vi "New One-Shot Subscription.vi"(10 "Ignore Past Updates? (F)":bool, 11 "OneShotSubscription In":refnum<class "OneShotSubscription.lvclass">) -> (3 "OneShotSubscription Out":refnum<class "OneShotSubscription.lvclass">)   [LabVIEW 2015, in "Mediator.lvlib" / "OneShotSubscription.lvclass"]
uses:
  OneShotSubscription.lvclass
  OneShotSubscription.lvclass/OneShotSubscription.ctl
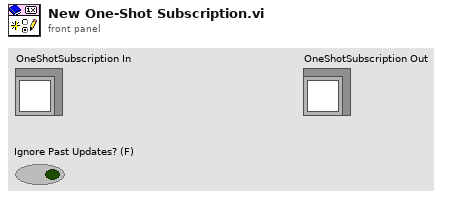
[diagram p1: front panel]
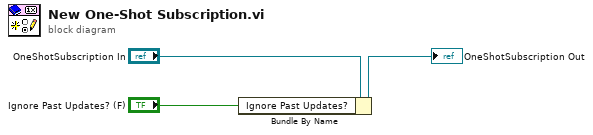
[diagram p0: block diagram]
diagram:
  n1 = Bundle By Name(cluster="OneShotSubscription In", "Ignore Past Updates?"="Ignore Past Updates? (F)") -> (→"OneShotSubscription Out":refnum<class "OneShotSubscription.lvclass">)
